vi "SERIAL_DecodeASCII.vi"(2 "navX Data":u8[](array[numeric]), 3 "Buffer":string) -> (0 "navX Data":u8[](array[numeric]), 1 "Valid?":bool)   [LabVIEW 2014, in "navX Library v1 (deprecated).lvlib"]
uses:
  navX Library v1 (deprecated).lvlib
  COMMON/TypeDefs/Value TypeDefs/navX Device Registers.ctl
  COMMON/TypeDefs/Value TypeDefs/navX NAVX_CAL_STATUS.ctl
  COMMON/Util/DataConvert/LabVIEW-to-navX/EncodeSignedHundredths.vi
  COMMON/Util/DataConvert/LabVIEW-to-navX/EncodeUnsignedHundredths.vi
  COMMON/Util/DataConvert/LabVIEW-to-navX/EncodeUnsignedThousandths.vi
  COMMON/Util/DataConvert/LabVIEW-to-navX/EncodeUInt8.vi
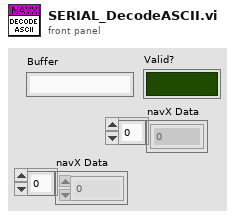
[diagram p1: front panel]
types:
  T1 = typedef "navX Library v1 (deprecated).lvlib/navX Device Registers.ctl" = u8
  T2 = typedef "navX Library v1 (deprecated).lvlib/navX NAVX_CAL_STATUS.ctl" = u8
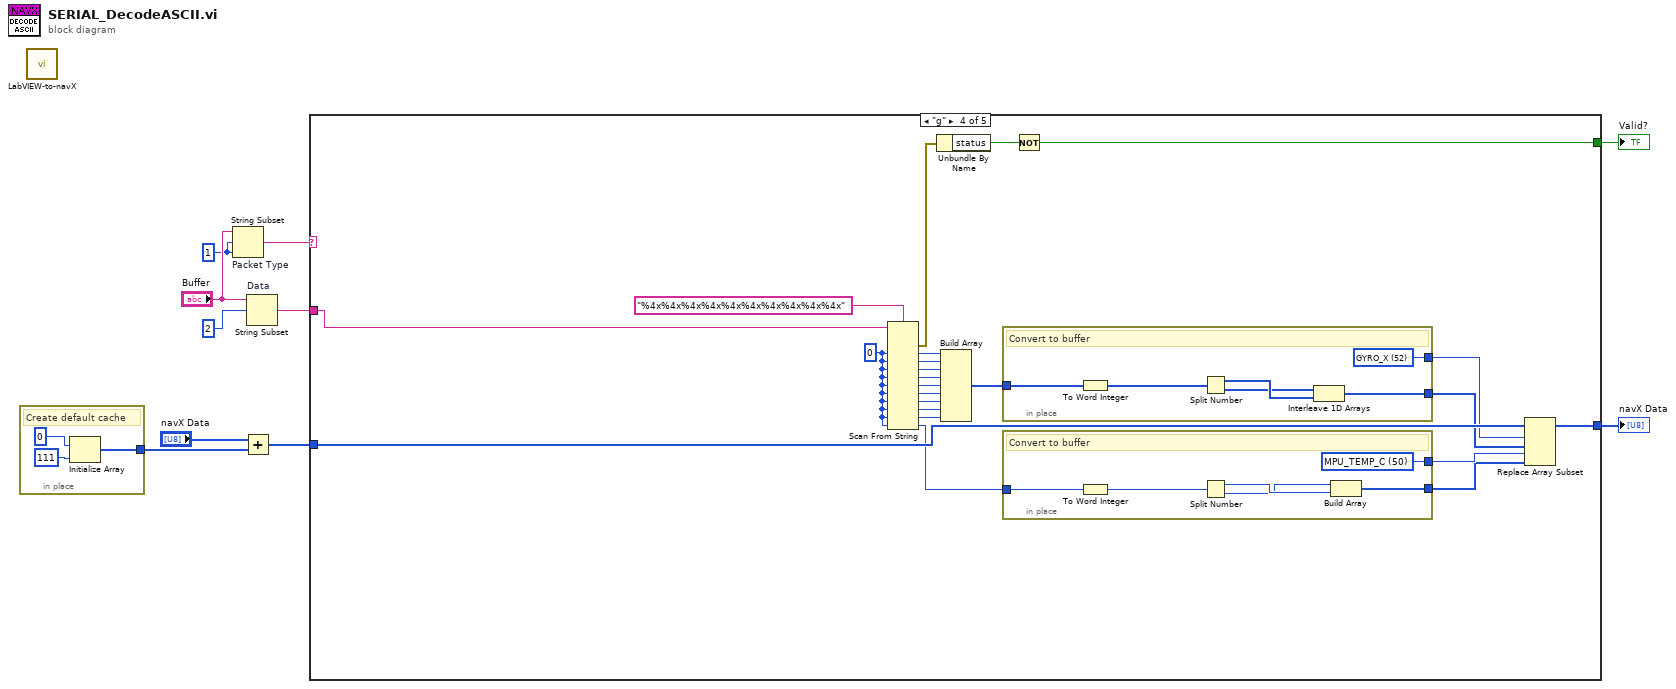
[diagram p0: block diagram]
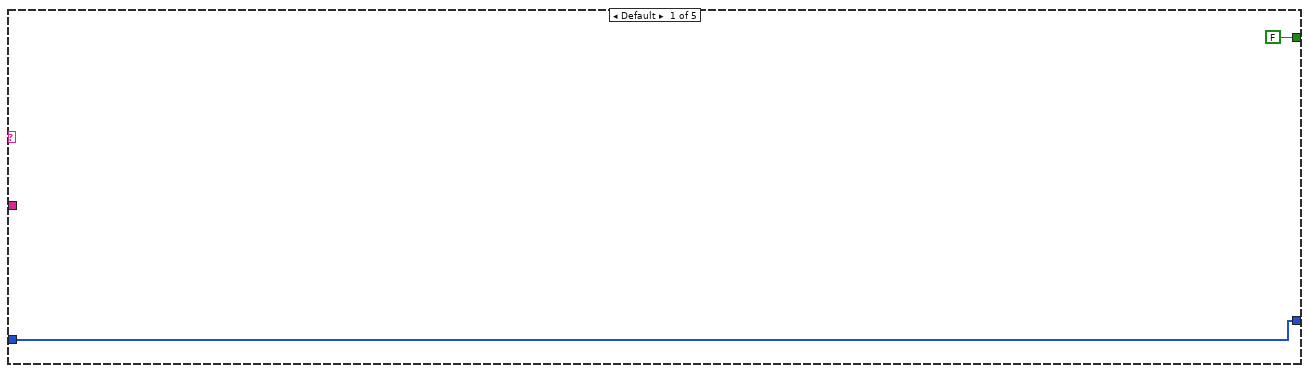
[diagram p2: hidden frame]
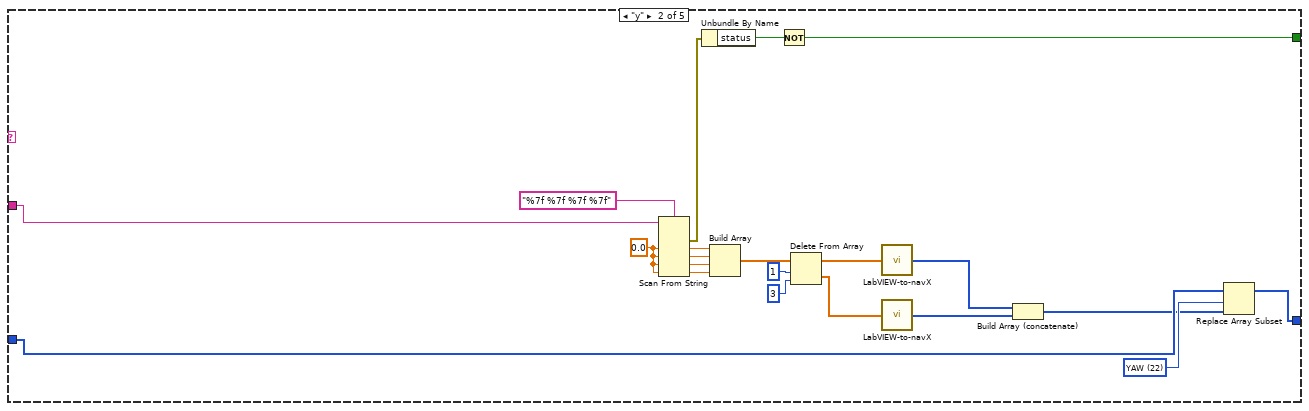
[diagram p3: hidden frame]
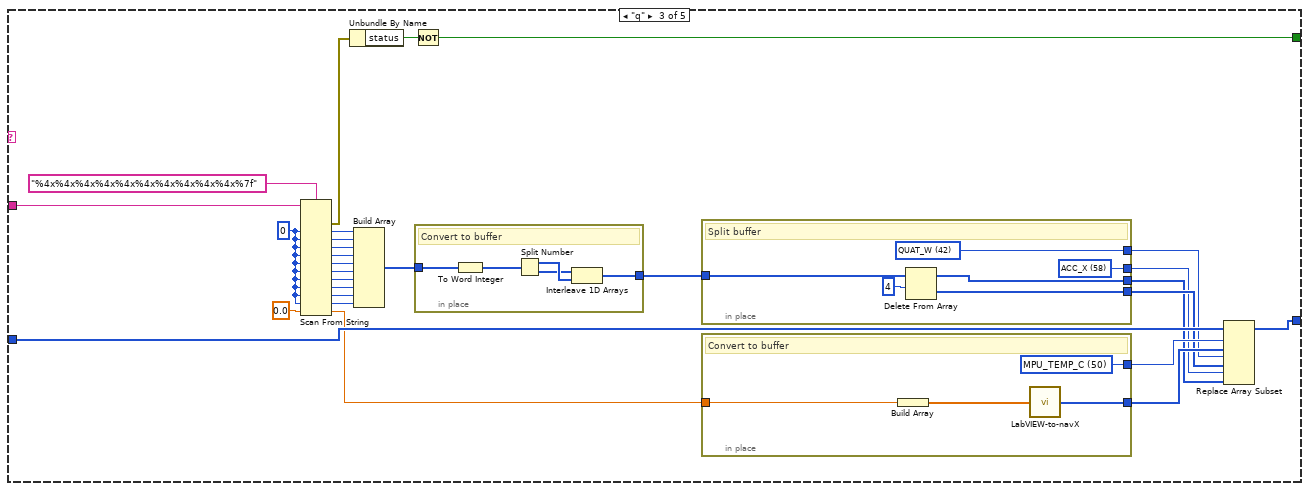
[diagram p4: hidden frame]
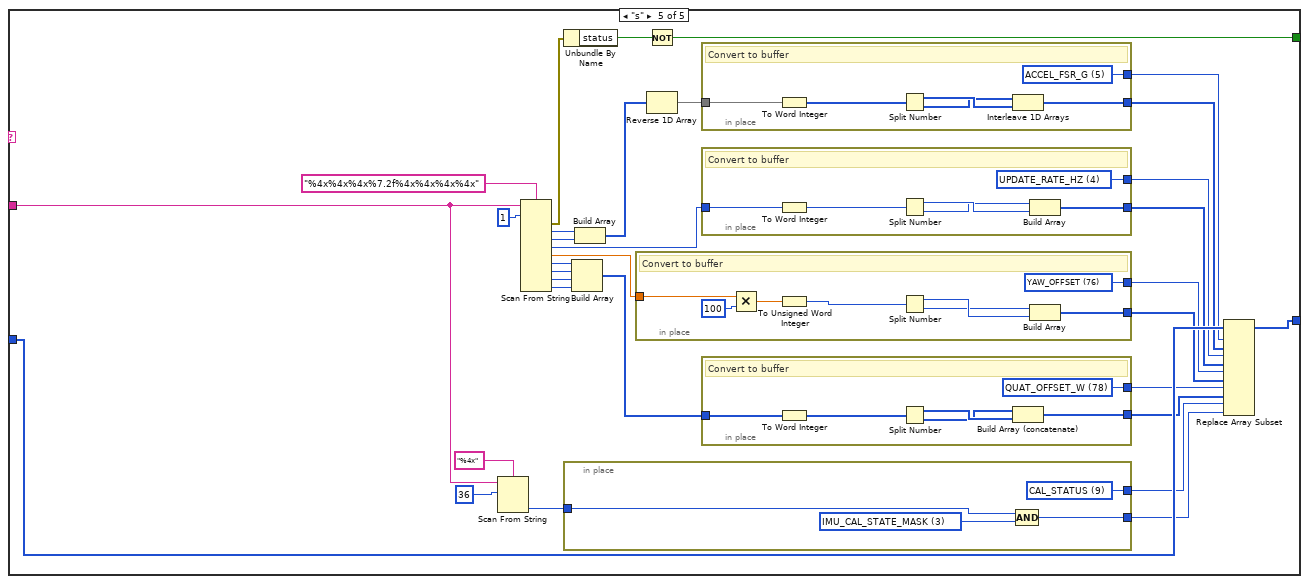
[diagram p5: hidden frame]
diagram:
  w8 = 1 ("offset (0)")
  n1 = in-place {
    in-place-border: [w11] -> w3
    # "Create default cache"
    n2 = Initialize Array(u8 0 ("Received Data"), u8 111 ("hex")) -> (w11:u8[])
  }
  n3 = call-poly "LabVIEW-to-navX.vi"() -> ()  [unwired: 1 in, 1 out]
  n4 = String Subset "Packet Type"(string="Buffer", offset (0)=w8, length (rest)=w8) -> (substring=w7:string)
  n5 = Add(x="navX Data", y=w3) -> (x+y=w2:u8[])
  n6 = String Subset "Data"(string="Buffer", offset (0)=2) -> (substring=w1:string)  [unwired: 1 in]
  n7 = case shown="\"g\"" w7 {
    tunnel: w1 -> [_ w35 w60 w80 w118]
    tunnel: w2 -> [w15 w29 w47 w91 w141]
    tunnel: [w15 w27 w46 w88 w142] -> w6
    tunnel: [FALSE w24 w48 w85 w143] -> w5
    frame Default {
    }
    frame "y" {
      w28 = T1 22 items=["WHOAMI"=0, "HW_REV"=1, "FW_VER_MAJOR"=2, "FW_VER_MINOR"=3, "UPDATE_RATE_HZ"=4, "ACCEL_FSR_G"=5, "GYRO_FSR_DPS"=6, "OP_STATUS"=8, "CAL_STATUS"=9, "SELFTEST_STATUS"=10, "CAPABILITY_FLAGS_L"=11, "CAPABILITY_FLAGS_H"=12, "SENSOR_STATUS"=16, "TIMESTAMP"=18, "YAW"=22, "PITCH"=24, "ROLL"=26, "HEADING"=28, "FUSED_HEADING"=30, "ALTITUDE_I"=32, "ALTITUDE_D"=34, "LINERA_ACC_X"=36, "LINERA_ACC_Y"=38, "LINERA_ACC_Z"=40, "QUAT_W"=42, "QUAT_X"=44, "QUAT_Y"=46, "QUAT_Z"=48, "MPU_TEMP_C"=50, "GYRO_X"=52, "GYRO_Y"=54, "GYRO_Z"=56, "ACC_X"=58, "ACC_Y"=60, "ACC_Z"=62, "MAG_X"=64, "MAG_Y"=66, "MAG_Z"=68, "PRESSURE_I"=70, "PRESSURE_D"=72, "PRESSURE_TEMP"=74, "YAW_OFFSET"=76, "QUAT_OFFSET_W"=78, "QUAT_OFFSET_X"=80, "QUAT_OFFSET_Y"=82, "QUAT_OFFSET_Z"=84, "INTEGRATION_CONTROL"=86, "VELOCITY_X"=88, "VELOCITY_Y"=92, "VELOCITY_Z"=96, "DISPLACMENT_X"=100, "DISPLACMENT_Y"=104, "DISPLACEMENT_Z"=108] ("Device Register")
      w34 = 0.0 ("default value 1")
      n8 = Scan From String(format string="%7f %7f %7f %7f", input string=w35, default 1=w34, default 2=w34, default 3=w34, default 4=w34) -> (error out=w26:errorcluster, output 1=w33:dbl, output 2=w30:dbl, output 3=w31:dbl, output 4=w32:dbl)  [unwired: 2 in, 2 out]
      n9 = Unbundle By Name(w26) -> ("status"=w25:bool)
      n10 = Build Array(w33, w30, w31, w32) -> (w19:dbl[])
      n11 = Not(x=w25) -> (.not. x?=w24:bool)
      n12 = Delete From Array(array=w19, length=1, index=3) -> (deleted portion=w21:dbl[], array with subset deleted=w20:dbl[])
      n13 = call-poly "LabVIEW-to-navX.vi"("Data In"=w20) -> ("Data Out"=w18:u8[])
      n14 = call-poly "LabVIEW-to-navX.vi"("Data In"=w21) -> ("Data Out"=w17:u8[])
      n15 = Build Array (concatenate)(w18, w17) -> (w16:u8[])
      n16 = Replace Array Subset(array=w29, new element=w16, index=w28) -> (w27:u8[])
    }
    frame "q" {
      w61 = u16 0 ("default value 1")
      n17 = Scan From String(format string="%4x%4x%4x%4x%4x%4x%4x%4x%4x%4x%7f", input string=w60, default 1=w61, default 2=w61, default 3=w61, default 4=w61, default 5=w61, default 6=w61, default 7=w61, default 8=w61, default 9=w61, default 10=w61, default 11=0.0 ("default value 11")) -> (error out=w62:errorcluster, output 1=w58:u16, output 2=w57:u16, output 3=w56:u16, output 4=w55:u16, output 5=w54:u16, output 6=w53:u16, output 7=w52:u16, output 8=w51:u16, output 9=w50:u16, output 10=w49:u16, output 11=w38:dbl)  [unwired: 2 in, 2 out]
      n18 = Unbundle By Name(w62) -> ("status"=w63:bool)
      n19 = Build Array(w58, w57, w56, w55, w54, w53, w52, w51, w50, w49) -> (w37:u16[])
      n20 = Not(x=w63) -> (.not. x?=w48:bool)
      n21 = in-place {
        in-place-border: w37 -> [w79]
        in-place-border: [w75] -> w43
        # "Convert to buffer"
        n22 = To Word Integer(number=w79) -> (16bit integer=w76:i16[])
        n23 = Split Number(x=w76) -> (hi(x)=w78:u8[], lo(x)=w77:u8[])
        n24 = Interleave 1D Arrays(w77, w78) -> (w75:u8[])
      }
      n25 = in-place {
        in-place-border: w43 -> [w70]
        in-place-border: [w68] -> w42
        in-place-border: [w67] -> w41
        in-place-border: [w66] -> w40
        in-place-border: [w65] -> w39
        w65 = T1 58 items=["WHOAMI"=0, "HW_REV"=1, "FW_VER_MAJOR"=2, "FW_VER_MINOR"=3, "UPDATE_RATE_HZ"=4, "ACCEL_FSR_G"=5, "GYRO_FSR_DPS"=6, "OP_STATUS"=8, "CAL_STATUS"=9, "SELFTEST_STATUS"=10, "CAPABILITY_FLAGS_L"=11, "CAPABILITY_FLAGS_H"=12, "SENSOR_STATUS"=16, "TIMESTAMP"=18, "YAW"=22, "PITCH"=24, "ROLL"=26, "HEADING"=28, "FUSED_HEADING"=30, "ALTITUDE_I"=32, "ALTITUDE_D"=34, "LINERA_ACC_X"=36, "LINERA_ACC_Y"=38, "LINERA_ACC_Z"=40, "QUAT_W"=42, "QUAT_X"=44, "QUAT_Y"=46, "QUAT_Z"=48, "MPU_TEMP_C"=50, "GYRO_X"=52, "GYRO_Y"=54, "GYRO_Z"=56, "ACC_X"=58, "ACC_Y"=60, "ACC_Z"=62, "MAG_X"=64, "MAG_Y"=66, "MAG_Z"=68, "PRESSURE_I"=70, "PRESSURE_D"=72, "PRESSURE_TEMP"=74, "YAW_OFFSET"=76, "QUAT_OFFSET_W"=78, "QUAT_OFFSET_X"=80, "QUAT_OFFSET_Y"=82, "QUAT_OFFSET_Z"=84, "INTEGRATION_CONTROL"=86, "VELOCITY_X"=88, "VELOCITY_Y"=92, "VELOCITY_Z"=96, "DISPLACMENT_X"=100, "DISPLACMENT_Y"=104, "DISPLACEMENT_Z"=108] ("Device Register")
        w67 = T1 42 items=["WHOAMI"=0, "HW_REV"=1, "FW_VER_MAJOR"=2, "FW_VER_MINOR"=3, "UPDATE_RATE_HZ"=4, "ACCEL_FSR_G"=5, "GYRO_FSR_DPS"=6, "OP_STATUS"=8, "CAL_STATUS"=9, "SELFTEST_STATUS"=10, "CAPABILITY_FLAGS_L"=11, "CAPABILITY_FLAGS_H"=12, "SENSOR_STATUS"=16, "TIMESTAMP"=18, "YAW"=22, "PITCH"=24, "ROLL"=26, "HEADING"=28, "FUSED_HEADING"=30, "ALTITUDE_I"=32, "ALTITUDE_D"=34, "LINERA_ACC_X"=36, "LINERA_ACC_Y"=38, "LINERA_ACC_Z"=40, "QUAT_W"=42, "QUAT_X"=44, "QUAT_Y"=46, "QUAT_Z"=48, "MPU_TEMP_C"=50, "GYRO_X"=52, "GYRO_Y"=54, "GYRO_Z"=56, "ACC_X"=58, "ACC_Y"=60, "ACC_Z"=62, "MAG_X"=64, "MAG_Y"=66, "MAG_Z"=68, "PRESSURE_I"=70, "PRESSURE_D"=72, "PRESSURE_TEMP"=74, "YAW_OFFSET"=76, "QUAT_OFFSET_W"=78, "QUAT_OFFSET_X"=80, "QUAT_OFFSET_Y"=82, "QUAT_OFFSET_Z"=84, "INTEGRATION_CONTROL"=86, "VELOCITY_X"=88, "VELOCITY_Y"=92, "VELOCITY_Z"=96, "DISPLACMENT_X"=100, "DISPLACMENT_Y"=104, "DISPLACEMENT_Z"=108] ("Device Register")
        # "Split buffer"
        n26 = Delete From Array(array=w70, length=4) -> (deleted portion=w68:u8[], array with subset deleted=w66:u8[])  [unwired: 1 in]
      }
      n27 = in-place {
        in-place-border: w38 -> [w72]
        in-place-border: [w71] -> w44
        in-place-border: [w74] -> w45
        w74 = T1 50 items=["WHOAMI"=0, "HW_REV"=1, "FW_VER_MAJOR"=2, "FW_VER_MINOR"=3, "UPDATE_RATE_HZ"=4, "ACCEL_FSR_G"=5, "GYRO_FSR_DPS"=6, "OP_STATUS"=8, "CAL_STATUS"=9, "SELFTEST_STATUS"=10, "CAPABILITY_FLAGS_L"=11, "CAPABILITY_FLAGS_H"=12, "SENSOR_STATUS"=16, "TIMESTAMP"=18, "YAW"=22, "PITCH"=24, "ROLL"=26, "HEADING"=28, "FUSED_HEADING"=30, "ALTITUDE_I"=32, "ALTITUDE_D"=34, "LINERA_ACC_X"=36, "LINERA_ACC_Y"=38, "LINERA_ACC_Z"=40, "QUAT_W"=42, "QUAT_X"=44, "QUAT_Y"=46, "QUAT_Z"=48, "MPU_TEMP_C"=50, "GYRO_X"=52, "GYRO_Y"=54, "GYRO_Z"=56, "ACC_X"=58, "ACC_Y"=60, "ACC_Z"=62, "MAG_X"=64, "MAG_Y"=66, "MAG_Z"=68, "PRESSURE_I"=70, "PRESSURE_D"=72, "PRESSURE_TEMP"=74, "YAW_OFFSET"=76, "QUAT_OFFSET_W"=78, "QUAT_OFFSET_X"=80, "QUAT_OFFSET_Y"=82, "QUAT_OFFSET_Z"=84, "INTEGRATION_CONTROL"=86, "VELOCITY_X"=88, "VELOCITY_Y"=92, "VELOCITY_Z"=96, "DISPLACMENT_X"=100, "DISPLACMENT_Y"=104, "DISPLACEMENT_Z"=108] ("Device Register")
        # "Convert to buffer"
        n28 = Build Array(w72) -> (w73:dbl[])
        n29 = call-poly "LabVIEW-to-navX.vi"("Data In"=w73) -> ("Data Out"=w71:u8[])
      }
      n30 = Replace Array Subset(array=w47, new element #1=w44, index #1=w45, new element #2=w42, index #2=w41, new element #3=w40, index #3=w39) -> (w46:u8[])
    }
    frame "g" {
      w81 = u16 0 ("default value 1")
      n31 = Scan From String(format string="%4x%4x%4x%4x%4x%4x%4x%4x%4x%4x", input string=w80, default 1=w81, default 2=w81, default 3=w81, default 4=w81, default 5=w81, default 6=w81, default 7=w81, default 8=w81, default 9=w81, default 10=w81) -> (error out=w86:errorcluster, output 1=w101:u16, output 2=w100:u16, output 3=w99:u16, output 4=w97:u16, output 5=w96:u16, output 6=w95:u16, output 7=w94:u16, output 8=w93:u16, output 9=w92:u16, output 10=w84:u16)  [unwired: 2 in, 2 out]
      n32 = Unbundle By Name(w86) -> ("status"=w87:bool)
      n33 = Build Array(w101, w100, w99, w97, w96, w95, w94, w93, w92) -> (w98:u16[])
      n34 = in-place {
        in-place-border: w98 -> [w114]
        in-place-border: [w110] -> w90
        in-place-border: [w109] -> w89
        w109 = T1 52 items=["WHOAMI"=0, "HW_REV"=1, "FW_VER_MAJOR"=2, "FW_VER_MINOR"=3, "UPDATE_RATE_HZ"=4, "ACCEL_FSR_G"=5, "GYRO_FSR_DPS"=6, "OP_STATUS"=8, "CAL_STATUS"=9, "SELFTEST_STATUS"=10, "CAPABILITY_FLAGS_L"=11, "CAPABILITY_FLAGS_H"=12, "SENSOR_STATUS"=16, "TIMESTAMP"=18, "YAW"=22, "PITCH"=24, "ROLL"=26, "HEADING"=28, "FUSED_HEADING"=30, "ALTITUDE_I"=32, "ALTITUDE_D"=34, "LINERA_ACC_X"=36, "LINERA_ACC_Y"=38, "LINERA_ACC_Z"=40, "QUAT_W"=42, "QUAT_X"=44, "QUAT_Y"=46, "QUAT_Z"=48, "MPU_TEMP_C"=50, "GYRO_X"=52, "GYRO_Y"=54, "GYRO_Z"=56, "ACC_X"=58, "ACC_Y"=60, "ACC_Z"=62, "MAG_X"=64, "MAG_Y"=66, "MAG_Z"=68, "PRESSURE_I"=70, "PRESSURE_D"=72, "PRESSURE_TEMP"=74, "YAW_OFFSET"=76, "QUAT_OFFSET_W"=78, "QUAT_OFFSET_X"=80, "QUAT_OFFSET_Y"=82, "QUAT_OFFSET_Z"=84, "INTEGRATION_CONTROL"=86, "VELOCITY_X"=88, "VELOCITY_Y"=92, "VELOCITY_Z"=96, "DISPLACMENT_X"=100, "DISPLACMENT_Y"=104, "DISPLACEMENT_Z"=108] ("Device Register")
        # "Convert to buffer"
        n35 = To Word Integer(number=w114) -> (16bit integer=w111:i16[])
        n36 = Split Number(x=w111) -> (hi(x)=w113:u8[], lo(x)=w112:u8[])
        n37 = Interleave 1D Arrays(w112, w113) -> (w110:u8[])
      }
      n38 = in-place {
        in-place-border: w84 -> [w104]
        in-place-border: [w106] -> w83
        in-place-border: [w105] -> w82
        w106 = T1 50 items=["WHOAMI"=0, "HW_REV"=1, "FW_VER_MAJOR"=2, "FW_VER_MINOR"=3, "UPDATE_RATE_HZ"=4, "ACCEL_FSR_G"=5, "GYRO_FSR_DPS"=6, "OP_STATUS"=8, "CAL_STATUS"=9, "SELFTEST_STATUS"=10, "CAPABILITY_FLAGS_L"=11, "CAPABILITY_FLAGS_H"=12, "SENSOR_STATUS"=16, "TIMESTAMP"=18, "YAW"=22, "PITCH"=24, "ROLL"=26, "HEADING"=28, "FUSED_HEADING"=30, "ALTITUDE_I"=32, "ALTITUDE_D"=34, "LINERA_ACC_X"=36, "LINERA_ACC_Y"=38, "LINERA_ACC_Z"=40, "QUAT_W"=42, "QUAT_X"=44, "QUAT_Y"=46, "QUAT_Z"=48, "MPU_TEMP_C"=50, "GYRO_X"=52, "GYRO_Y"=54, "GYRO_Z"=56, "ACC_X"=58, "ACC_Y"=60, "ACC_Z"=62, "MAG_X"=64, "MAG_Y"=66, "MAG_Z"=68, "PRESSURE_I"=70, "PRESSURE_D"=72, "PRESSURE_TEMP"=74, "YAW_OFFSET"=76, "QUAT_OFFSET_W"=78, "QUAT_OFFSET_X"=80, "QUAT_OFFSET_Y"=82, "QUAT_OFFSET_Z"=84, "INTEGRATION_CONTROL"=86, "VELOCITY_X"=88, "VELOCITY_Y"=92, "VELOCITY_Z"=96, "DISPLACMENT_X"=100, "DISPLACMENT_Y"=104, "DISPLACEMENT_Z"=108] ("Device Register")
        # "Convert to buffer"
        n39 = To Word Integer(number=w104) -> (16bit integer=w103:i16)
        n40 = Split Number(x=w103) -> (hi(x)=w108:u8, lo(x)=w107:u8)
        n41 = Build Array(w107, w108) -> (w105:u8[])
      }
      n42 = Not(x=w87) -> (.not. x?=w85:bool)
      n43 = Replace Array Subset(array=w91, new element #1=w90, index #1=w89, new element #2=w82, index #2=w83) -> (w88:u8[])
    }
    frame "s" {
      n44 = Scan From String(format string="%4x", input string=w118, initial scan location=u32 36) -> (output 1=w116:u32)  [unwired: 2 in, 3 out]
      n45 = Scan From String(format string="%4x%4x%4x%7.2f%4x%4x%4x%4x", input string=w118, initial scan location=u32 1) -> (error out=w144:errorcluster, output 1=w140:u32, output 2=w139:u32, output 3=w134:u32, output 4=w131:dbl, output 5=w128:u32, output 6=w127:u32, output 7=w126:u32, output 8=w125:u32)  [unwired: 9 in, 2 out]
      n46 = Unbundle By Name(w144) -> ("status"=w145:bool)
      n47 = in-place {
        in-place-border: w116 -> [w149]
        in-place-border: [w148] -> w121
        in-place-border: [w147] -> w120
        w148 = T1 9 items=["WHOAMI"=0, "HW_REV"=1, "FW_VER_MAJOR"=2, "FW_VER_MINOR"=3, "UPDATE_RATE_HZ"=4, "ACCEL_FSR_G"=5, "GYRO_FSR_DPS"=6, "OP_STATUS"=8, "CAL_STATUS"=9, "SELFTEST_STATUS"=10, "CAPABILITY_FLAGS_L"=11, "CAPABILITY_FLAGS_H"=12, "SENSOR_STATUS"=16, "TIMESTAMP"=18, "YAW"=22, "PITCH"=24, "ROLL"=26, "HEADING"=28, "FUSED_HEADING"=30, "ALTITUDE_I"=32, "ALTITUDE_D"=34, "LINERA_ACC_X"=36, "LINERA_ACC_Y"=38, "LINERA_ACC_Z"=40, "QUAT_W"=42, "QUAT_X"=44, "QUAT_Y"=46, "QUAT_Z"=48, "MPU_TEMP_C"=50, "GYRO_X"=52, "GYRO_Y"=54, "GYRO_Z"=56, "ACC_X"=58, "ACC_Y"=60, "ACC_Z"=62, "MAG_X"=64, "MAG_Y"=66, "MAG_Z"=68, "PRESSURE_I"=70, "PRESSURE_D"=72, "PRESSURE_TEMP"=74, "YAW_OFFSET"=76, "QUAT_OFFSET_W"=78, "QUAT_OFFSET_X"=80, "QUAT_OFFSET_Y"=82, "QUAT_OFFSET_Z"=84, "INTEGRATION_CONTROL"=86, "VELOCITY_X"=88, "VELOCITY_Y"=92, "VELOCITY_Z"=96, "DISPLACMENT_X"=100, "DISPLACMENT_Y"=104, "DISPLACEMENT_Z"=108] ("Device Register")
        w150 = T2 3 items=["IMU_CAL_STATE_MASK"=3, "IMU_CAL_INPROGRESS"=0, "IMU_CAL_ACCUMULATE"=1, "IMU_CAL_COMPLETE"=2, "MAG_CAL_COMPLETE"=4, "BARO_CAL_COMPLETE"=8] ("NAVX_CAL_STATUS")
        n48 = Compound Arithmetic op=AND(w149, w150) -> (w147:u32)
      }
      n49 = Build Array(w128, w127, w126, w125) -> (w124:u32[])
      n50 = Build Array(w140, w139) -> (w138:u32[])
      n51 = in-place {
        in-place-border: w131 -> [w161]
        in-place-border: [w158] -> w129
        in-place-border: [w157] -> w130
        w157 = T1 76 items=["WHOAMI"=0, "HW_REV"=1, "FW_VER_MAJOR"=2, "FW_VER_MINOR"=3, "UPDATE_RATE_HZ"=4, "ACCEL_FSR_G"=5, "GYRO_FSR_DPS"=6, "OP_STATUS"=8, "CAL_STATUS"=9, "SELFTEST_STATUS"=10, "CAPABILITY_FLAGS_L"=11, "CAPABILITY_FLAGS_H"=12, "SENSOR_STATUS"=16, "TIMESTAMP"=18, "YAW"=22, "PITCH"=24, "ROLL"=26, "HEADING"=28, "FUSED_HEADING"=30, "ALTITUDE_I"=32, "ALTITUDE_D"=34, "LINERA_ACC_X"=36, "LINERA_ACC_Y"=38, "LINERA_ACC_Z"=40, "QUAT_W"=42, "QUAT_X"=44, "QUAT_Y"=46, "QUAT_Z"=48, "MPU_TEMP_C"=50, "GYRO_X"=52, "GYRO_Y"=54, "GYRO_Z"=56, "ACC_X"=58, "ACC_Y"=60, "ACC_Z"=62, "MAG_X"=64, "MAG_Y"=66, "MAG_Z"=68, "PRESSURE_I"=70, "PRESSURE_D"=72, "PRESSURE_TEMP"=74, "YAW_OFFSET"=76, "QUAT_OFFSET_W"=78, "QUAT_OFFSET_X"=80, "QUAT_OFFSET_Y"=82, "QUAT_OFFSET_Z"=84, "INTEGRATION_CONTROL"=86, "VELOCITY_X"=88, "VELOCITY_Y"=92, "VELOCITY_Z"=96, "DISPLACMENT_X"=100, "DISPLACMENT_Y"=104, "DISPLACEMENT_Z"=108] ("Device Register")
        # "Convert to buffer"
        n52 = Multiply(x=w161, y=u16 100) -> (x*y=w160:dbl)
        n53 = To Unsigned Word Integer(number=w160) -> (unsigned 16bit integer=w159:u16)
        n54 = Split Number(x=w159) -> (hi(x)=w163:u8, lo(x)=w162:u8)
        n55 = Build Array(w162, w163) -> (w158:u8[])
      }
      n56 = Not(x=w145) -> (.not. x?=w143:bool)
      n57 = Reverse 1D Array(array=w138) -> (reversed array=w137:u32[])
      n58 = in-place {
        in-place-border: w137 -> [w176]
        in-place-border: [w172] -> w135
        in-place-border: [w171] -> w136
        w171 = T1 5 items=["WHOAMI"=0, "HW_REV"=1, "FW_VER_MAJOR"=2, "FW_VER_MINOR"=3, "UPDATE_RATE_HZ"=4, "ACCEL_FSR_G"=5, "GYRO_FSR_DPS"=6, "OP_STATUS"=8, "CAL_STATUS"=9, "SELFTEST_STATUS"=10, "CAPABILITY_FLAGS_L"=11, "CAPABILITY_FLAGS_H"=12, "SENSOR_STATUS"=16, "TIMESTAMP"=18, "YAW"=22, "PITCH"=24, "ROLL"=26, "HEADING"=28, "FUSED_HEADING"=30, "ALTITUDE_I"=32, "ALTITUDE_D"=34, "LINERA_ACC_X"=36, "LINERA_ACC_Y"=38, "LINERA_ACC_Z"=40, "QUAT_W"=42, "QUAT_X"=44, "QUAT_Y"=46, "QUAT_Z"=48, "MPU_TEMP_C"=50, "GYRO_X"=52, "GYRO_Y"=54, "GYRO_Z"=56, "ACC_X"=58, "ACC_Y"=60, "ACC_Z"=62, "MAG_X"=64, "MAG_Y"=66, "MAG_Z"=68, "PRESSURE_I"=70, "PRESSURE_D"=72, "PRESSURE_TEMP"=74, "YAW_OFFSET"=76, "QUAT_OFFSET_W"=78, "QUAT_OFFSET_X"=80, "QUAT_OFFSET_Y"=82, "QUAT_OFFSET_Z"=84, "INTEGRATION_CONTROL"=86, "VELOCITY_X"=88, "VELOCITY_Y"=92, "VELOCITY_Z"=96, "DISPLACMENT_X"=100, "DISPLACMENT_Y"=104, "DISPLACEMENT_Z"=108] ("Device Register")
        # "Convert to buffer"
        n59 = To Word Integer(number=w176) -> (16bit integer=w173:i16[])
        n60 = Split Number(x=w173) -> (hi(x)=w175:u8[], lo(x)=w174:u8[])
        n61 = Interleave 1D Arrays(w174, w175) -> (w172:u8[])
      }
      n62 = in-place {
        in-place-border: w134 -> [w170]
        in-place-border: [w166] -> w132
        in-place-border: [w165] -> w133
        w165 = T1 4 items=["WHOAMI"=0, "HW_REV"=1, "FW_VER_MAJOR"=2, "FW_VER_MINOR"=3, "UPDATE_RATE_HZ"=4, "ACCEL_FSR_G"=5, "GYRO_FSR_DPS"=6, "OP_STATUS"=8, "CAL_STATUS"=9, "SELFTEST_STATUS"=10, "CAPABILITY_FLAGS_L"=11, "CAPABILITY_FLAGS_H"=12, "SENSOR_STATUS"=16, "TIMESTAMP"=18, "YAW"=22, "PITCH"=24, "ROLL"=26, "HEADING"=28, "FUSED_HEADING"=30, "ALTITUDE_I"=32, "ALTITUDE_D"=34, "LINERA_ACC_X"=36, "LINERA_ACC_Y"=38, "LINERA_ACC_Z"=40, "QUAT_W"=42, "QUAT_X"=44, "QUAT_Y"=46, "QUAT_Z"=48, "MPU_TEMP_C"=50, "GYRO_X"=52, "GYRO_Y"=54, "GYRO_Z"=56, "ACC_X"=58, "ACC_Y"=60, "ACC_Z"=62, "MAG_X"=64, "MAG_Y"=66, "MAG_Z"=68, "PRESSURE_I"=70, "PRESSURE_D"=72, "PRESSURE_TEMP"=74, "YAW_OFFSET"=76, "QUAT_OFFSET_W"=78, "QUAT_OFFSET_X"=80, "QUAT_OFFSET_Y"=82, "QUAT_OFFSET_Z"=84, "INTEGRATION_CONTROL"=86, "VELOCITY_X"=88, "VELOCITY_Y"=92, "VELOCITY_Z"=96, "DISPLACMENT_X"=100, "DISPLACMENT_Y"=104, "DISPLACEMENT_Z"=108] ("Device Register")
        # "Convert to buffer"
        n63 = To Word Integer(number=w170) -> (16bit integer=w167:i16)
        n64 = Split Number(x=w167) -> (hi(x)=w169:u8, lo(x)=w168:u8)
        n65 = Build Array(w168, w169) -> (w166:u8[])
      }
      n66 = in-place {
        in-place-border: w124 -> [w156]
        in-place-border: [w152] -> w122
        in-place-border: [w151] -> w123
        w151 = T1 78 items=["WHOAMI"=0, "HW_REV"=1, "FW_VER_MAJOR"=2, "FW_VER_MINOR"=3, "UPDATE_RATE_HZ"=4, "ACCEL_FSR_G"=5, "GYRO_FSR_DPS"=6, "OP_STATUS"=8, "CAL_STATUS"=9, "SELFTEST_STATUS"=10, "CAPABILITY_FLAGS_L"=11, "CAPABILITY_FLAGS_H"=12, "SENSOR_STATUS"=16, "TIMESTAMP"=18, "YAW"=22, "PITCH"=24, "ROLL"=26, "HEADING"=28, "FUSED_HEADING"=30, "ALTITUDE_I"=32, "ALTITUDE_D"=34, "LINERA_ACC_X"=36, "LINERA_ACC_Y"=38, "LINERA_ACC_Z"=40, "QUAT_W"=42, "QUAT_X"=44, "QUAT_Y"=46, "QUAT_Z"=48, "MPU_TEMP_C"=50, "GYRO_X"=52, "GYRO_Y"=54, "GYRO_Z"=56, "ACC_X"=58, "ACC_Y"=60, "ACC_Z"=62, "MAG_X"=64, "MAG_Y"=66, "MAG_Z"=68, "PRESSURE_I"=70, "PRESSURE_D"=72, "PRESSURE_TEMP"=74, "YAW_OFFSET"=76, "QUAT_OFFSET_W"=78, "QUAT_OFFSET_X"=80, "QUAT_OFFSET_Y"=82, "QUAT_OFFSET_Z"=84, "INTEGRATION_CONTROL"=86, "VELOCITY_X"=88, "VELOCITY_Y"=92, "VELOCITY_Z"=96, "DISPLACMENT_X"=100, "DISPLACMENT_Y"=104, "DISPLACEMENT_Z"=108] ("Device Register")
        # "Convert to buffer"
        n67 = To Word Integer(number=w156) -> (16bit integer=w153:i16[])
        n68 = Split Number(x=w153) -> (hi(x)=w155:u8[], lo(x)=w154:u8[])
        n69 = Build Array (concatenate)(w154, w155) -> (w152:u8[])
      }
      n70 = Replace Array Subset(array=w141, new element #1=w135, index #1=w136, new element #2=w132, index #2=w133, new element #3=w129, index #3=w130, new element #4=w122, index #4=w123, new element #5=w120, index #5=w121) -> (w142:u8[])
    }
  }
  "Valid?" <- w5
  "navX Data" <- w6
